vi "Launch Async Process.vi"(8 "error in (no error)":errorcluster, 11 "MQTT_Base in":refnum<class "MQTT_Base.lvclass">) -> ()   [LabVIEW 2013, in "MQTT Base.lvlib" / "MQTT_Base.lvclass"]
uses:
  MQTT_Base.lvclass
  MQTT_Base.lvclass/MQTT_Base.ctl
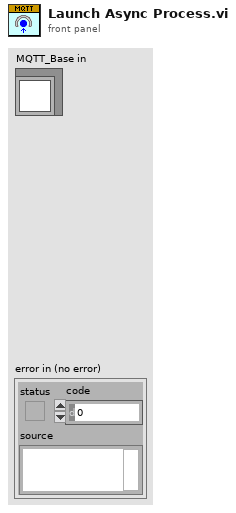
[diagram p1: front panel]
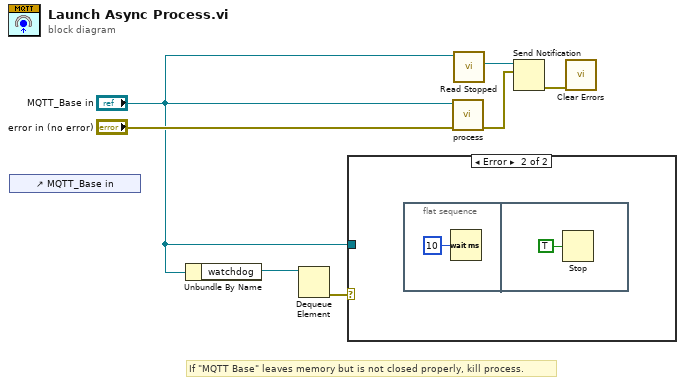
[diagram p0: block diagram]
diagram:
  # "If \"MQTT Base\" leaves memory but is not closed properly, kill process."
  n1 = control-ref of="MQTT_Base in"() -> ()  [unwired: 1 out]
  n2 = Unbundle By Name("MQTT_Base in") -> ("watchdog"=w6:refnum<queue>)
  n3 = Dequeue Element(queue=w6) -> (error out=w5:errorcluster)  [unwired: 2 in, 3 out]
  n4 = case shown="Error" w5 {
    tunnel: "MQTT_Base in" -> [_ _]
    frame No Error {
    }
    frame Error {
      n5 = flat-sequence {
        frame #0 {
          n6 = Wait (ms)(milliseconds to wait=u32 10) -> ()  [unwired: 1 out]
        }
        frame #1 {
          n7 = Stop(stop? (T)=TRUE) -> ()
        }
      }
    }
  }
  n8 = call-dynamic "process.vi"("error in (no error)"="error in (no error)", "MQTT_Base in"="MQTT_Base in") -> ("error out"=w3:errorcluster)  [unwired: 9 in]
  n9 = call "Read Stopped.vi"("MQTT_Base in"="MQTT_Base in") -> ("Stopped"=w4:refnum<notifier>)  [unwired: 8 in, 2 out]
  n10 = Send Notification(notification=w3, notifier=w4) -> (error out=w1:errorcluster)  [unwired: 1 in, 1 out]
  n11 = call <vilib>:"Clear Errors.vi"("error in (no error)"=w1) -> ()  [unwired: 6 in, 1 out]
